vi "UpdateExpLog.vi"(8 "error in (no error)":errorcluster) -> (0 "error out":errorcluster)   [LabVIEW 2019]
uses:
  controls/GlobalExp.vi
  Global.lvlib
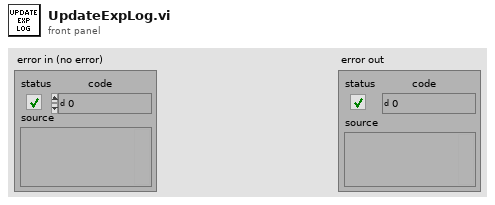
[diagram p1: front panel]
types:
  T1 = typedef "MasterExpControl.ctl" = cluster{"Main Steps":dbl, "Main Runs":dbl, "ExpStatus":enum16{"Innit", "Stop", "Idle", "MainRunning", "AuxRunning"}, "Main Current Step":dbl, "ExpNum":dbl, "NewData":bool, "date":string, "command":string, "Stop":bool, "Pause":bool, "Mathematica":string, "Main/Meta":bool, "UpdateMath":bool, "Camera":bool, "MetaExpOver":bool, "NextMetaExp":bool}
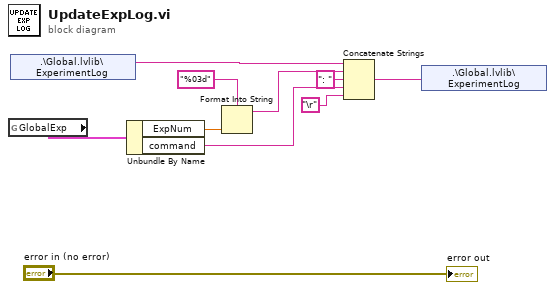
[diagram p0: block diagram]
diagram:
  n1 = global read "GlobalExp.vi" "GlobalExp"() -> (w9:T1)
  n2 = shared-variable ".\\Global.lvlib\\ExperimentLog"() -> (w8:string)  [unwired: 1 in, 1 out]
  n3 = Unbundle By Name(w9) -> ("ExpNum"=w7:dbl, "command"=w3:string)
  n4 = Format Into String(format string="%03d", w7) -> (resulting string=w6:string)  [unwired: 2 in, 1 out]
  n5 = Concatenate Strings(w8, w6, ": " ("string"), w3, "\r") -> (w2:string)
  n6 = shared-variable ".\\Global.lvlib\\ExperimentLog"(w2) -> ()  [unwired: 1 in, 1 out]
  "error out" <- "error in (no error)"
